vi "Upgrade Version.vi"(8 "error in (no error)":errorcluster, 10 "New Version":string, 11 "Device Item Ref In in":T1 format="%.0x") -> (0 "error out":errorcluster, 3 "Device Item Ref In out":T1 format="%.0x")   [LabVIEW 2018, in "NI-XNET Monitor System Explorer.lvlib"]
uses:
  NI-XNET Monitor System Explorer.lvlib
  <vilib>/NI Veristand/Custom Device API/Custom Device Item Ref.ctl
  Shared/Constants.vi
  <vilib>/NI Veristand/Custom Device API/Get Item Property (String).vi
  Shared/NI-XNET Monitor Shared.lvlib
  <vilib>/NI Veristand/Custom Device API/Custom Device API.lvlib
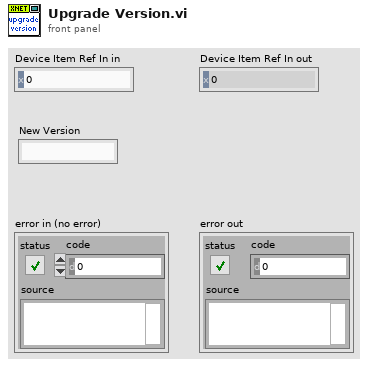
[diagram p1: front panel]
types:
  T1 = typedef "Custom Device API.lvlib/Custom Device Item Ref.ctl" = u64
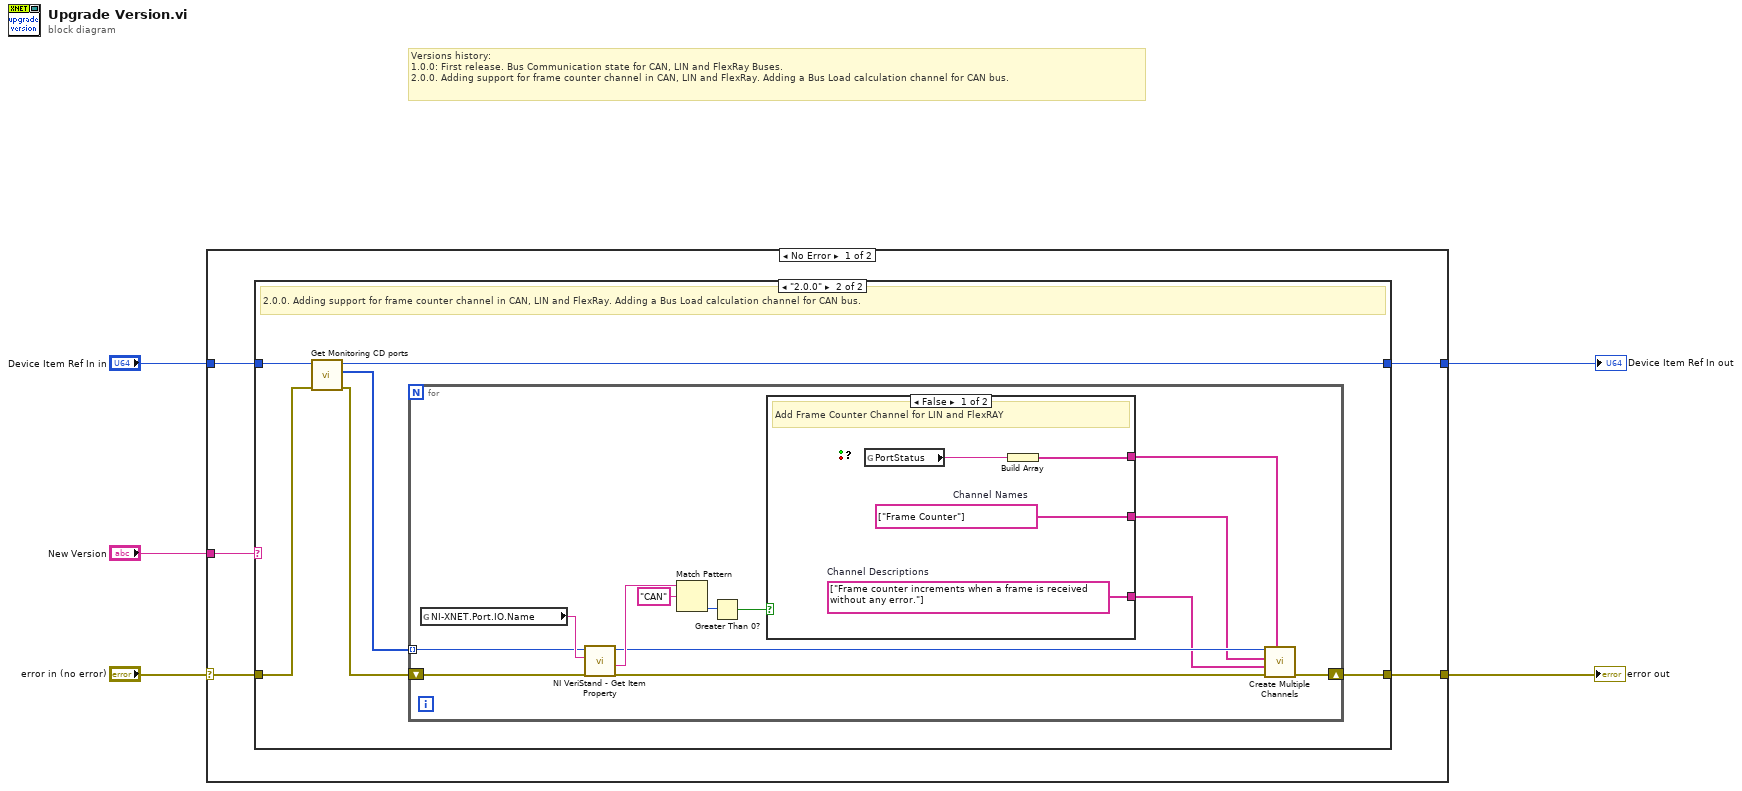
[diagram p0: block diagram]
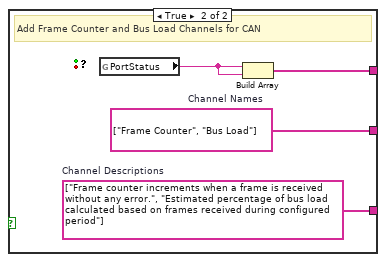
[diagram p3: hidden frame]
diagram:
  # "Versions history:\n1.0.0: First release. Bus Communication state for CAN, LIN and FlexRay Buses.\n2.0.0. Adding support for frame counter channel in CAN, LIN and FlexRay. Adding a Bus Load calculation channel for CAN bus."
  n1 = case shown="No Error" "error in (no error)" {
    selector: "error in (no error)" -> [w6 w40]
    tunnel: "Device Item Ref In in" -> [w8 w41]
    tunnel: [w9 w41] -> w3
    tunnel: [w7 w40] -> w2
    tunnel: "New Version" -> [w10 _]
    frame No Error {
      n2 = case shown="\"2.0.0\"" w10 {
        tunnel: [w12 w16] -> w9
        tunnel: w8 -> [w12 w18]
        tunnel: [w11 w13] -> w7
        tunnel: w6 -> [w11 w17]
        frame Default {
        }
        frame "2.0.0" {
          # "2.0.0. Adding support for frame counter channel in CAN, LIN and FlexRay. Adding a Bus Load calculation channel for CAN bus."
          n3 = call "Get Monitoring CD ports.vi"("Error In"=w17, "Device Item Ref in"=w18) -> ("Error Out"=w14:errorcluster, "CD Port Refs"=w15:T1[], "Device Item Ref out"=w16:T1)  [unwired: 6 in, 1 out]
          n4 = for {
            tunnel: w15 -> [w28] mode=indexing
            shift-right: [w25] -> w13
            shift-left: w14 -> [w27]
            n5 = global read "Constants.vi" "NI-XNET.Port.IO.Name"() -> (w31:string)
            n6 = call-poly <vilib>:"NI VeriStand - Get Item Property.vi"("error in (no error)"=w27, "Property Name"=w31, "Item Ref in"=w28) -> ("error out"=w22:errorcluster, "Value"=w26:string, "Item Ref out"=w23:T1)  [unwired: 5 in, 1 out]
            n7 = Match Pattern(string=w26, regular expression="CAN") -> (offset past match=w30:i32)  [unwired: 1 in, 3 out]
            n8 = Greater Than 0?(x=w30) -> (x > 0?=w24:bool)
            n9 = case shown="False" w24 {
              tunnel: [w33 w38] -> w21
              tunnel: [w34 w37] -> w20
              tunnel: [w32 w36] -> w19
              frame False {
                w32 = string[] ["Frame counter increments when a frame is received without any error."]  # Channel Descriptions
                w33 = string[] ["Frame Counter"]  # Channel Names
                # "Add Frame Counter Channel for LIN and FlexRAY"
                n10 = global read "Constants.vi" "PortStatus"() -> (w35:string)
                n11 = Build Array(w35) -> (w34:string[])
              }
              frame True {
                w36 = string[] ["Frame counter increments when a frame is received without any error.", "Estimated percentage of bus load calculated based on frames received during configured period"]  # Channel Descriptions
                w38 = string[] ["Frame Counter", "Bus Load"]  # Channel Names
                # "Add Frame Counter and Bus Load Channels for CAN"
                n12 = global read "Constants.vi" "PortStatus"() -> (w39:string)
                n13 = Build Array(w39, w39) -> (w37:string[])
              }
            }
            n14 = call "Create Multiple Channels.vi"("Icons"=w20, "error in"=w22, "Channel Descriptions"=w19, "Channel Names"=w21, "Item Ref in"=w23) -> ("error out"=w25:errorcluster)  [unwired: 6 in]
          }
        }
      }
    }
    frame Error {
    }
  }
  "error out" <- w2
  "Device Item Ref In out" <- w3
